vi "ExAppCamera.vi"() -> ()   [LabVIEW 2010]
uses:
  GlobalCamOpen.vi
  GlobalCCDMaxDim.vi
  GlobalInitializeFlag.vi
  GlobalFramesToStr.vi
  GlobalTimingMode.vi
  GlobalAcquireFocusFlag.vi
  GlobalExposure.vi
  GlobalUserBin.vi
  GlobalBin2x.vi
  GlobalFullBin.vi
  GlobalFlipFlag.vi
  GlobalReverseFlag.vi
  GlobalIBackImgHndl.vi
  GlobalIFlatImgHndl.vi
panel:
  out "Camera Opened":bool
  in  "Exit program":bool
  out "error out":errorcluster
  in  "error in (no error)":errorcluster
  in  "Tab Control":T1(tab)
  in  "Focus/Acquire Mode":u32=1 min=1 max=5 step=1
  in  "Number of Frames to store":u32=1 min=1 step=1
  in  "Intensifier":bool
  in  "Readout Port":i32=-1 min=-1 step=1
  in  "ADC Offset 2":i32=-1 min=-1 step=1
  in  "ADC Gain 2":i32=-1 min=-1 step=1
  in  "ADC speed":i32=-2 min=-3 step=1
  in  "Trigger Edge":u32(ring)=1 items=["N/A", "Positive (leading) edge", "Negative (falling) edge"]
  in  "Timing Mode":u32(ring)=1 items=["N/A", "Free Run/Timed", "Trigger First (PM only)", "Ext Sync/Strobed ", "Variable Exp (PM only)", "Flash Mode (PM only)"]
  out "Pixel Time":i32
  out "Bit Depth":i32
  out "ReadOut port":i32
  out "ADC Offset":i32
  out "ADC Gain":i32
  out "ADC Speed":i32
  in  "Set Experiment \nParameters, Initialize \nCamera/Controller":bool
  out "temperature":dbl format="%.2f"
  out "Temperature Read":dbl(slide) scale=-120.0..20.0
  in  "Temperature":dbl format="%.2f"
  in  "Exposure":dbl format="%.2f"
  out "Controller Initialized":bool
  out "Total":u32
  out "Y dim":u32
  out "X dim":u32
  in  "Y Bin":u32=1 min=1 step=1
  in  "Y End":u32=100 min=1 step=1
  in  "Y Start":u32=1 min=1 step=1
  in  "X Bin":u32=1 min=1 step=1
  in  "X End":u32=100 min=1 step=1
  in  "X Start":u32=1 min=1 step=1
  out "Bin 2":bool
  out "User":bool
  out "Full":bool
  in  "Binned by 2 Button":bool
  in  "User Defined Button":bool
  in  "Full CCD Button":bool
  out "Flip\nActive":bool
  in  "Flip flag Button":bool
  out "Reverse\nActive":bool
  in  "Image Reverse Button":bool
  out "Flat Field\nActive":bool
  out "Background \nActive":bool
  in  "Frame number to read":u32=1 min=1 step=1
  in  "Flat Button":bool
  in  "Back Button":bool
  in  "Full File Name":path
  in  "FileType":u32=67371008
  out "Reverse\nactive":bool
  out "Flip\nactive":bool
  out "Flat Field\nactive":bool
  out "background\nactive":bool
  in  "Reverse\nbutton":bool
  in  "Flip\nbutton":bool
  in  "Flat Field\nbutton":bool
  in  "Background\nbutton":bool
  in  "stop 2":bool
  in  "Start":bool
  out "Camera initialized":bool
  in  "Full File Name\nfor Acqure":path
  in  "OK Button":bool
  out "camera initialized":bool
  # "Note: In order for any parameters to change and be downloaded the initialize button must be hit."
  # "The following are read \nfrom camera after setting\nvalues to left.\n-1 value means it isn't \nsupported by camera."
  # "For Slowest ADC speed set this to -3\nFor Fastest ADC speed set this to -2\nTo use current ADC speed don't  hook up or use -1\notherwise put speed in as kHz"
  # "To use current gain don't hook up or set to -1"
  # "To use current gain don't hook up or set to -1"
  # "To use current gain don't hook up or set to -1"
  # "NOTE: if background subtraction and/or flat field are set, there are no \nchecks in this example for changes to the ROI."
  # "Pixels coming back\nfrom Camera"
  # "File Types:\nSPE = 67371008\nTIF   = 67174400\nPMI  = 67436544"
  # "Browse match pattern is set to *.spe.  Modify this if different file type is needed."
  # "Instructions:\nMake sure camera/controller has been initialized.  LED should be ON.\nPress \"Start Data collection\" button (a display should appear).\nWhen done press the \"STOP\" button (the display should disappear).\nLive Operation buttons only work while collecting data (not before)\nTo setup Live Operations before, go to Live Operations tab."
  # "Live Operations\n(will only work while collecting data)."
  # "Instructions:\nMake sure the camera/controller has been initialized (the light should be on).\nMake sure to put in a file name with path to save data.\nPress 'Start' button and display will pop up and data will be saved in file."
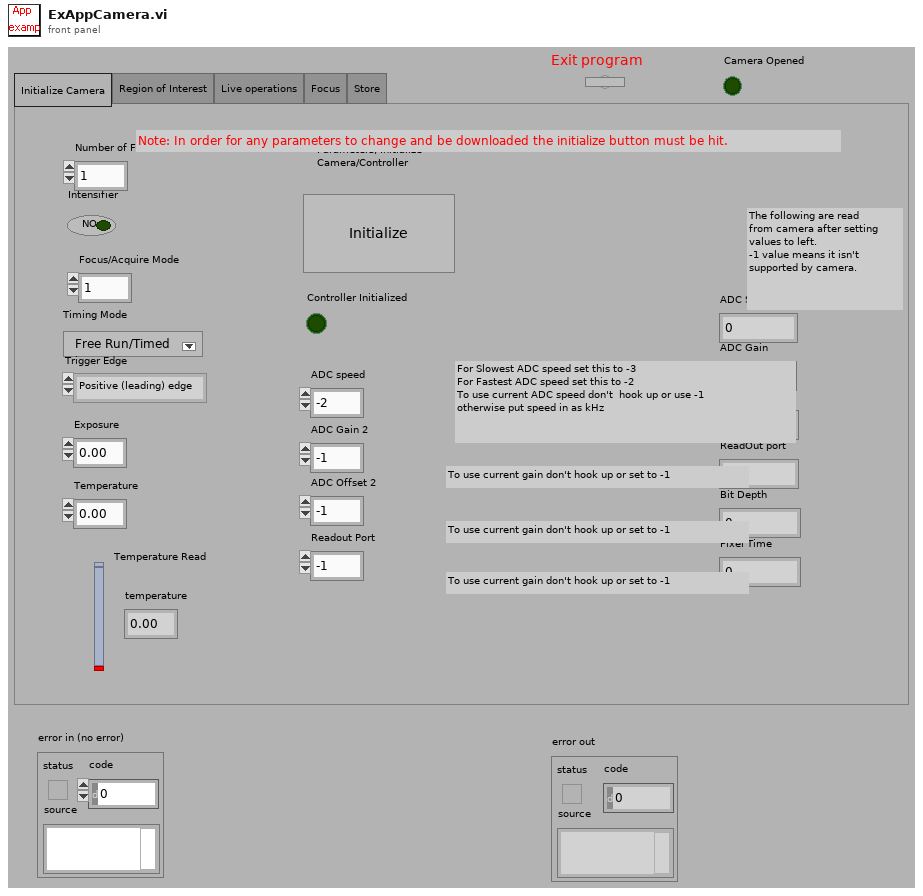
[diagram p1: front panel]
types:
  T1 = enum32{"Initialize Camera", "Region of Interest", "Live operations", "Focus", "Store"}
  T2 = cluster{"X Start":u32, "X End":u32, "X Bin":u32, "Y Start":u32, "Y End":u32, "Y Bin":u32}
  T3 = cluster{i32, "CCD Max X":u32, i32, i32, "CCD Max Y":u32, i32}
  T4 = cluster{"Camera Handle":u32, "Pulser Handle":u32, "File Handle":u32, "Display Handle":u32, "Image Handle":u32}
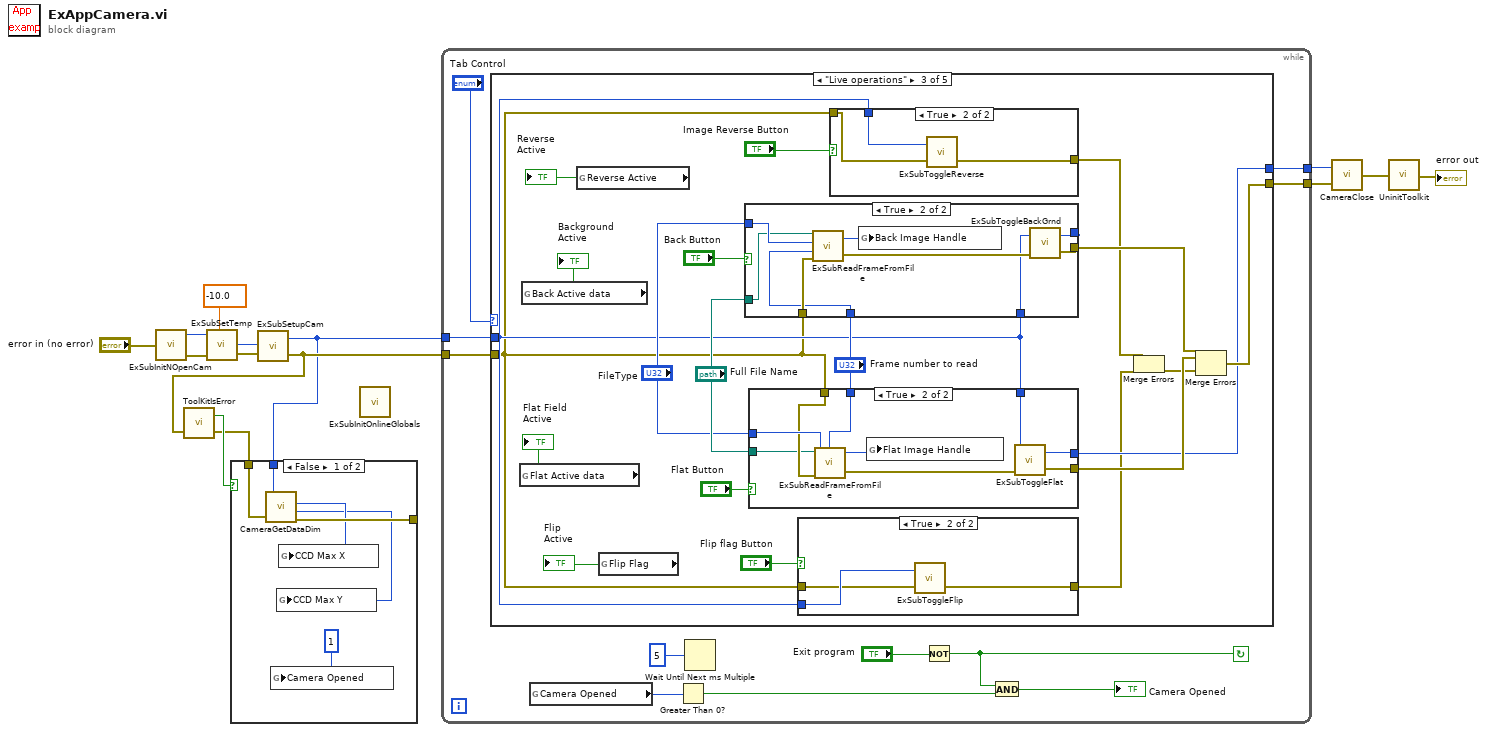
[diagram p0: block diagram]
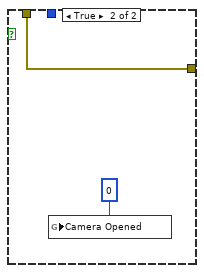
[diagram p2: hidden frame]
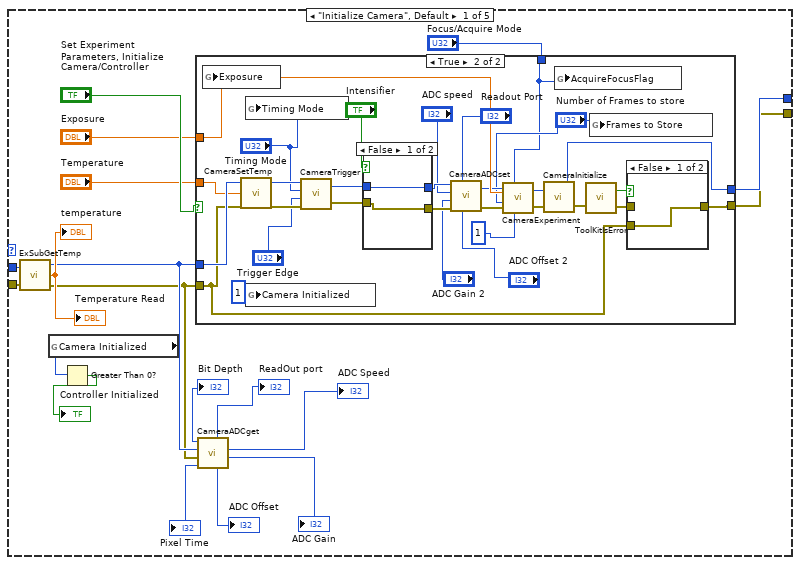
[diagram p3: hidden frame]
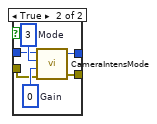
[diagram p6: hidden frame]
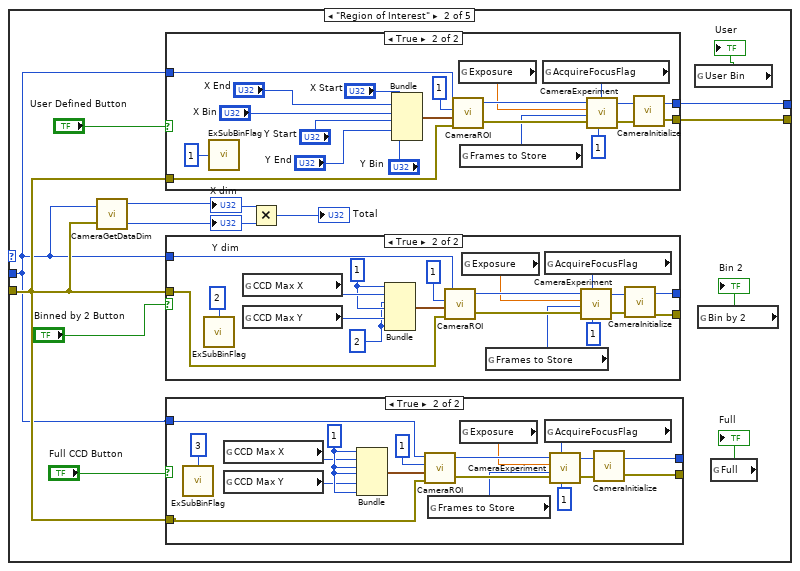
[diagram p7: hidden frame]
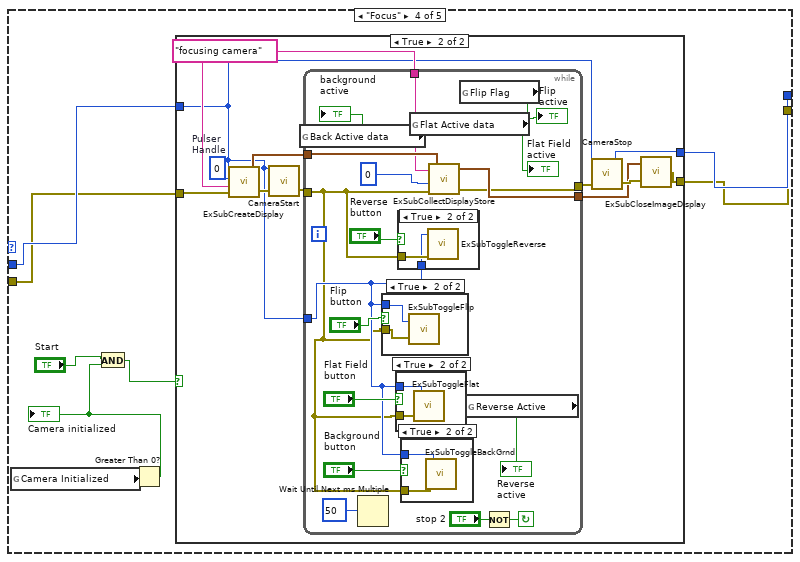
[diagram p15: hidden frame]
diagram:
  n1 = call "ExSubInitNOpenCam.vi"("error in (no error)"="error in (no error)") -> ("Camera Handle"=w12:u32, "error out"=w13:errorcluster)
  n2 = call "ExSubSetTemp.vi"("error in (no error)"=w13, "Temperature"=-10.0, "CameraHandle"=w12) -> ("error out"=w10:errorcluster, "Camera Handle"=w3:u32)
  n3 = call "ExSubSetupCam.vi"("error in (no error)"=w10, "Camera Handle"=w3) -> ("error out"=w4:errorcluster, "Camera Handle"=w2:u32)
  n4 = call <userlib>:"ToolKitIsError.vi"("error in"=w4) -> ("error out"=w1:errorcluster, "Error Flag"=w5:bool)  [unwired: 1 in]
  n5 = case shown="False" w5 {
    tunnel: w1 -> [w18 w22]
    tunnel: [w19 w22] -> _
    tunnel: w2 -> [w15 _]
    frame False {
      n6 = call <userlib>:"CameraGetDataDim.vi"("Camera Handle"=w15, "error in"=w18) -> ("Xdim"=w17:u32, "Ydim"=w16:u32, "error out"=w19:errorcluster)  [unwired: 1 out]
      n7 = global write "GlobalCamOpen.vi" "Camera Opened"(1) -> ()
      n8 = global write "GlobalCCDMaxDim.vi" "CCD Max Y"(w16) -> ()
      n9 = global write "GlobalCCDMaxDim.vi" "CCD Max X"(w17) -> ()
    }
    frame True {
      n10 = global write "GlobalCamOpen.vi" "Camera Opened"(0) -> ()
    }
  }
  n11 = call "ExSubInitOnlineGlobals.vi"() -> ()  [unwired: 1 in]
  n12 = while {
    tunnel: w2 -> [w33]
    tunnel: w4 -> [w30]
    tunnel: [w29] -> w9
    tunnel: [w28] -> w8
    stop <- w26 continue-if-true
    n13 = case shown="\"Live operations\"" "Tab Control" {
      tunnel: w33 -> [w52 w100 w176 w223 w273]
      tunnel: w30 -> [w44 w101 w175 w222 w272]
      tunnel: [w36 w99 w183 w225 w270] -> w29
      tunnel: [w35 w98 w184 w224 w271] -> w28
      frame "Initialize Camera", Default {
        n14 = call "ExSubGetTemp.vi"("Camera Handle"=w52, "error in (no error)"=w44) -> ("Camera Handle"=w43:u32, "Actual Temperature"=→"temperature" →"Temperature Read":dbl, "error out"=w42:errorcluster)
        n15 = global read "GlobalInitializeFlag.vi" "Camera Initialized"() -> (w47:u32)
        n16 = Greater Than 0?(x=w47) -> (x > 0?=→"Controller Initialized":bool)
        n17 = case shown="True" "Set Experiment \nParameters, Initialize \nCamera/Controller" {
          tunnel: "Exposure" -> [_ w73]
          tunnel: "Temperature" -> [_ w82]
          tunnel: w42 -> [w53 w57]
          tunnel: w43 -> [w54 w83]
          tunnel: [w53 w60] -> w35
          tunnel: [w54 w58] -> w36
          tunnel: "Focus/Acquire Mode" -> [_ w55]
          frame False {
          }
          frame True {
            n18 = global write "GlobalExposure.vi" "Exposure"(w73) -> ()
            n19 = call <userlib>:"CameraSetTemp.vi"("error in (no error)"=w57, "Temperature"=w82, "Camera Handle"=w83) -> ("error out"=w72:errorcluster, "Camera Handle"=w71:u32)
            n20 = global write "GlobalTimingMode.vi" "Timing Mode"("Timing Mode") -> ()
            n21 = global write "GlobalInitializeFlag.vi" "Camera Initialized"(1) -> ()
            n22 = call <userlib>:"CameraTrigger.vi"("error in"=w72, "Trigger Edge"="Trigger Edge", "Timing Mode"="Timing Mode", "Camera Handle"=w71) -> ("error out"=w68:errorcluster, "Camera Handle"=w69:u32)
            n23 = case shown="False" "Intensifier" {
              tunnel: [w88 w94] -> w79
              tunnel: [w87 w93] -> w80
              tunnel: w69 -> [w88 w90]
              tunnel: w68 -> [w87 w89]
              frame False {
              }
              frame True {
                w91 = u32 0  # Gain
                w92 = u32 3  # Mode
                n24 = call <userlib>:"CameraIntensMode.vi"("error in"=w89, "Intensifier Gain"=w91, "Mode"=w92, "Camera Handle"=w90) -> ("error out"=w93:errorcluster, "Camera Handle"=w94:u32)
              }
            }
            n25 = call <userlib>:"CameraADCset.vi"("ADC offset"="ADC Offset 2", "Read Out port"="Readout Port", "error in (no error)"=w80, "ADC Gain"="ADC Gain 2", "ADC Speed"="ADC speed", "Camera Handle"=w79) -> ("error out"=w66:errorcluster, "Camera Handle"=w65:u32)
            n26 = call <userlib>:"CameraExperiment.vi"("Number of Accumulations"=1, "Acquire / Focus Flag"=w55, "error in"=w66, "Number of Images"="Number of Frames to store", "Exposure (sec)"=w73, "Camera Handle"=w65) -> ("error out"=w64:errorcluster, "Camera Handle"=w63:u32)
            n27 = call <userlib>:"CameraInitialize.vi"("error in"=w64, "Camera Handle"=w63) -> ("error out"=w59:errorcluster, "Camera Handle"=w58:u32)
            n28 = global write "GlobalAcquireFocusFlag.vi" "AcquireFocusFlag"(w55) -> ()
            n29 = call <userlib>:"ToolKitIsError.vi"("error in"=w59) -> ("error out"=w61:errorcluster, "Error Flag"=w62:bool)  [unwired: 1 in]
            n30 = global write "GlobalFramesToStr.vi" "Frames to Store"("Number of Frames to store") -> ()
            n31 = case shown="False" w62 {
              tunnel: w61 -> [_ w86]
              tunnel: [w85 w86] -> w60
              tunnel: w57 -> [w85 _]
              frame False {
              }
              frame True {
              }
            }
          }
        }
        n32 = call <userlib>:"CameraADCget.vi"("Camera handle"=w43, "error in (no error)"=w42) -> ("Bit Depth"=→"Bit Depth":i32, "Pixel Time"=→"Pixel Time":i32, "Readout Port"=→"ReadOut port":i32, "ADC Offset"=→"ADC Offset":i32, "ADC Speed"=→"ADC Speed":i32, "ADC Gain"=→"ADC Gain":i32)  [unwired: 2 out]
      }
      frame "Region of Interest" {
        n33 = call <userlib>:"CameraGetDataDim.vi"("Camera Handle"=w100, "error in"=w101) -> ("Xdim"=w97:u32, "Ydim"=w96:u32)  [unwired: 2 out]
        "X dim" <- w97
        "Y dim" <- w96
        n34 = case shown="True" "User Defined Button" {
          tunnel: w100 -> [w150 w154]
          tunnel: [w150 w169] -> w99
          tunnel: w101 -> [w149 w153]
          tunnel: [w149 w166] -> w98
          frame False {
          }
          frame True {
            n35 = call "ExSubBinFlag.vi"("Binning \nUser = 1\nBin 2 = 2\nFull = 3"=1) -> ()
            n36 = Bundle("X Start"="X Start", "X End"="X End", "X Bin"="X Bin", "Y Start"="Y Start", "Y End"="Y End", "Y Bin"="Y Bin") -> (w155:T2)  [unwired: 1 in]
            n37 = call <userlib>:"CameraROI.vi"("error in"=w153, "ROI Params"=w155, "ROI Index"=1, "Camera Handle"=w154) -> ("error out"=w168:errorcluster, "Camera Handle"=w171:u32)
            n38 = global read "GlobalExposure.vi" "Exposure"() -> (w164:dbl)
            n39 = global read "GlobalFramesToStr.vi" "Frames to Store"() -> (w163:u32)
            n40 = global read "GlobalAcquireFocusFlag.vi" "AcquireFocusFlag"() -> (w162:u32)
            n41 = call <userlib>:"CameraExperiment.vi"("Number of Accumulations"=1, "Acquire / Focus Flag"=w162, "error in"=w168, "Number of Images"=w163, "Exposure (sec)"=w164, "Camera Handle"=w171) -> ("error out"=w167:errorcluster, "Camera Handle"=w170:u32)
            n42 = call <userlib>:"CameraInitialize.vi"("error in"=w167, "Camera Handle"=w170) -> ("error out"=w166:errorcluster, "Camera Handle"=w169:u32)
          }
        }
        n43 = case shown="True" "Binned by 2 Button" {
          tunnel: w100 -> [w129 w134]
          tunnel: [w129 w140] -> _
          tunnel: w101 -> [w128 w135]
          tunnel: [w128 w139] -> _
          frame False {
          }
          frame True {
            w131 = 2
            w132 = 1
            n44 = call "ExSubBinFlag.vi"("Binning \nUser = 1\nBin 2 = 2\nFull = 3"=2) -> ()
            n45 = global read "GlobalCCDMaxDim.vi" "CCD Max X"() -> (w138:u32)
            n46 = global read "GlobalCCDMaxDim.vi" "CCD Max Y"() -> (w137:u32)
            n47 = Bundle(w132, "CCD Max X"=w138, w131, w132, "CCD Max Y"=w137, w131) -> (w136:T3)  [unwired: 1 in]
            n48 = call <userlib>:"CameraROI.vi"("error in"=w135, "ROI Params"=w136, "ROI Index"=1, "Camera Handle"=w134) -> ("error out"=w146:errorcluster, "Camera Handle"=w148:u32)
            n49 = global read "GlobalExposure.vi" "Exposure"() -> (w143:dbl)
            n50 = global read "GlobalFramesToStr.vi" "Frames to Store"() -> (w142:u32)
            n51 = global read "GlobalAcquireFocusFlag.vi" "AcquireFocusFlag"() -> (w141:u32)
            n52 = call <userlib>:"CameraExperiment.vi"("Number of Accumulations"=1, "Acquire / Focus Flag"=w141, "error in"=w146, "Number of Images"=w142, "Exposure (sec)"=w143, "Camera Handle"=w148) -> ("error out"=w145:errorcluster, "Camera Handle"=w147:u32)
            n53 = call <userlib>:"CameraInitialize.vi"("error in"=w145, "Camera Handle"=w147) -> ("error out"=w139:errorcluster, "Camera Handle"=w140:u32)
          }
        }
        n54 = case shown="True" "Full CCD Button" {
          tunnel: w100 -> [w109 w112]
          tunnel: [w109 w119] -> _
          tunnel: w101 -> [w108 w111]
          tunnel: [w108 w118] -> _
          frame False {
          }
          frame True {
            w117 = 1
            n55 = call "ExSubBinFlag.vi"("Binning \nUser = 1\nBin 2 = 2\nFull = 3"=3) -> ()
            n56 = global read "GlobalCCDMaxDim.vi" "CCD Max X"() -> (w116:u32)
            n57 = global read "GlobalCCDMaxDim.vi" "CCD Max Y"() -> (w115:u32)
            n58 = Bundle(w117, "CCD Max X"=w116, w117, w117, "CCD Max Y"=w115, w117) -> (w114:T3)  [unwired: 1 in]
            n59 = call <userlib>:"CameraROI.vi"("error in"=w111, "ROI Params"=w114, "ROI Index"=1, "Camera Handle"=w112) -> ("error out"=w125:errorcluster, "Camera Handle"=w127:u32)
            n60 = global read "GlobalFramesToStr.vi" "Frames to Store"() -> (w121:u32)
            n61 = global read "GlobalExposure.vi" "Exposure"() -> (w122:dbl)
            n62 = global read "GlobalAcquireFocusFlag.vi" "AcquireFocusFlag"() -> (w120:u32)
            n63 = call <userlib>:"CameraExperiment.vi"("Number of Accumulations"=1, "Acquire / Focus Flag"=w120, "error in"=w125, "Number of Images"=w121, "Exposure (sec)"=w122, "Camera Handle"=w127) -> ("error out"=w124:errorcluster, "Camera Handle"=w126:u32)
            n64 = call <userlib>:"CameraInitialize.vi"("error in"=w124, "Camera Handle"=w126) -> ("error out"=w118:errorcluster, "Camera Handle"=w119:u32)
          }
        }
        n65 = Multiply(x=w97, y=w96) -> (x*y=→"Total":u32)
        n66 = global read "GlobalUserBin.vi" "User Bin"() -> (→"User":bool)
        n67 = global read "GlobalBin2x.vi" "Bin by 2"() -> (→"Bin 2":bool)
        n68 = global read "GlobalFullBin.vi" "Full"() -> (→"Full":bool)
      }
      frame "Live operations" {
        n69 = global read "GlobalIFlatImgHndl.vi" "Flat Active data"() -> (→"Flat Field\nActive":bool)
        n70 = global read "GlobalIBackImgHndl.vi" "Back Active data"() -> (→"Background \nActive":bool)
        n71 = global read "GlobalReverseFlag.vi" "Reverse Active"() -> (→"Reverse\nActive":bool)
        n72 = global read "GlobalFlipFlag.vi" "Flip Flag"() -> (→"Flip\nActive":bool)
        n73 = case shown="True" "Back Button" {
          tunnel: "Full File Name" -> [_ w219]
          tunnel: "FileType" -> [_ w220]
          tunnel: w175 -> [w212 w221]
          tunnel: [w212 w215] -> w186
          tunnel: "Frame number to read" -> [_ w218]
          tunnel: w176 -> [w211 w214]
          tunnel: [w211 w213] -> _
          frame False {
          }
          frame True {
            n74 = call "ExSubReadFrameFromFile.vi"("error in (no error)"=w221, "Frame to pull off"=w218, "File type"=w220, "path to file to open"=w219) -> ("error out"=w216:errorcluster, "Image Handle"=w217:u32)
            n75 = global write "GlobalIBackImgHndl.vi" "Back Image Handle"(w217) -> ()
            n76 = call "ExSubToggleBackGrnd.vi"("error in (no error)"=w216, "Camera Handle"=w214) -> ("error out"=w215:errorcluster, "Camera Handle"=w213:u32)
          }
        }
        n77 = case shown="True" "Flat Button" {
          tunnel: "Full File Name" -> [_ w207]
          tunnel: "FileType" -> [_ w210]
          tunnel: w175 -> [w201 w208]
          tunnel: [w201 w203] -> w185
          tunnel: "Frame number to read" -> [_ w209]
          tunnel: w176 -> [w200 w205]
          tunnel: [w200 w204] -> w183
          frame False {
          }
          frame True {
            n78 = call "ExSubReadFrameFromFile.vi"("error in (no error)"=w208, "Frame to pull off"=w209, "File type"=w210, "path to file to open"=w207) -> ("error out"=w202:errorcluster, "Image Handle"=w206:u32)
            n79 = global write "GlobalIFlatImgHndl.vi" "Flat Image Handle"(w206) -> ()
            n80 = call "ExSubToggleFlat.vi"("error in (no error)"=w202, "Camera Handle"=w205) -> ("error out"=w203:errorcluster, "Camera Handle"=w204:u32)
          }
        }
        n81 = case shown="True" "Flip flag Button" {
          tunnel: w176 -> [_ w199]
          tunnel: w175 -> [w196 w198]
          tunnel: [w196 w197] -> w174
          frame False {
          }
          frame True {
            n82 = call "ExSubToggleFlip.vi"("error in (no error)"=w198, "Camera Handle"=w199) -> ("error out"=w197:errorcluster)  [unwired: 1 out]
          }
        }
        n83 = case shown="True" "Image Reverse Button" {
          tunnel: w176 -> [_ w194]
          tunnel: w175 -> [w192 w195]
          tunnel: [w192 w193] -> w173
          frame False {
          }
          frame True {
            n84 = call "ExSubToggleReverse.vi"("error in (no error)"=w195, "Camera Handle"=w194) -> ("error out"=w193:errorcluster)  [unwired: 1 out]
          }
        }
        n85 = Merge Errors(w173, w174) -> (w172:errorcluster)
        n86 = Merge Errors(w186, w185, w172) -> (w184:errorcluster)
      }
      frame "Focus" {
        n87 = global read "GlobalInitializeFlag.vi" "Camera Initialized"() -> (w227:u32)
        n88 = Greater Than 0?(x=w227) -> (x > 0?=w226:bool)
        "Camera initialized" <- w226
        n89 = And(x="Start", y=w226) -> (x .and. y?=w229:bool)
        n90 = case shown="True" w229 {
          tunnel: w222 -> [w230 w239]
          tunnel: w223 -> [w231 w232]
          tunnel: [w231 w236] -> w225
          tunnel: [w230 w235] -> w224
          frame False {
          }
          frame True {
            w233 = "focusing camera"
            w240 = u32 0  # Pulser  Handle
            n91 = call "ExSubCreateDisplay.vi"("error in (no error)"=w239, "File and Display Name"=w233, "Pulser Handle"=w240, "Camera Handle"=w232) -> ("error out"=w241:errorcluster, "Handles Out"=w243:T4)
            n92 = call <userlib>:"CameraStart.vi"("error in"=w241, "Camera Handle"=w232) -> ("error out"=w242:errorcluster)  [unwired: 1 out]
            n93 = while {
              tunnel: w243 -> [w260]
              tunnel: w242 -> [w248]
              tunnel: [w258] -> w238
              tunnel: [w259] -> w234
              tunnel: w233 -> [w254]
              tunnel: w232 -> [w249]
              stop <- w256 continue-if-true
              n94 = global read "GlobalIBackImgHndl.vi" "Back Active data"() -> (→"background\nactive":bool)
              n95 = Wait Until Next ms Multiple(millisecond multiple=u32 50) -> ()  [unwired: 1 out]
              n96 = case shown="True" "Flip\nbutton" {
                tunnel: w249 -> [_ w266]
                tunnel: w248 -> [_ w267]
                frame False {
                }
                frame True {
                  n97 = call "ExSubToggleFlip.vi"("error in (no error)"=w267, "Camera Handle"=w266) -> ()  [unwired: 2 out]
                }
              }
              n98 = case shown="True" "Flat Field\nbutton" {
                tunnel: w249 -> [_ w264]
                tunnel: w248 -> [_ w265]
                frame False {
                }
                frame True {
                  n99 = call "ExSubToggleFlat.vi"("error in (no error)"=w265, "Camera Handle"=w264) -> ()  [unwired: 2 out]
                }
              }
              n100 = case shown="True" "Reverse\nbutton" {
                tunnel: w248 -> [_ w269]
                tunnel: w249 -> [_ w268]
                frame False {
                }
                frame True {
                  n101 = call "ExSubToggleReverse.vi"("error in (no error)"=w269, "Camera Handle"=w268) -> ()  [unwired: 2 out]
                }
              }
              n102 = case shown="True" "Background\nbutton" {
                tunnel: w249 -> [_ w263]
                tunnel: w248 -> [_ w262]
                frame False {
                }
                frame True {
                  n103 = call "ExSubToggleBackGrnd.vi"("error in (no error)"=w262, "Camera Handle"=w263) -> ()  [unwired: 2 out]
                }
              }
              n104 = global read "GlobalIFlatImgHndl.vi" "Flat Active data"() -> (→"Flat Field\nactive":bool)
              n105 = call "ExSubCollectDisplayStore.vi"("error in (no error)"=w248, "Store flag"=0, "Display Title"=w254, "Handle Cluster"=w260) -> ("error out"=w258:errorcluster, "Handle Cluster Out"=w259:T4)  [unwired: 1 out]
              n106 = global read "GlobalFlipFlag.vi" "Flip Flag"() -> (→"Flip\nactive":bool)
              n107 = global read "GlobalReverseFlag.vi" "Reverse Active"() -> (→"Reverse\nactive":bool)
              n108 = Not(x="stop 2") -> (.not. x?=w256:bool)
            }
            n109 = call <userlib>:"CameraStop.vi"("error in"=w238, "Camera Handle"=w232) -> ("error out"=w237:errorcluster, "Camera Handle"=w236:u32)
            n110 = call "ExSubCloseImageDisplay.vi"("error in (no error)"=w237, "Handles In"=w234) -> ("error out"=w235:errorcluster)
          }
        }
      }
      frame "Store" {
        n111 = global read "GlobalInitializeFlag.vi" "Camera Initialized"() -> (w275:u32)
        n112 = Greater Than 0?(x=w275) -> (x > 0?=w274:bool)
        "camera initialized" <- w274
        n113 = And(x="OK Button", y=w274) -> (x .and. y?=w277:bool)
        n114 = case shown="True" w277 {
          tunnel: w273 -> [w279 w288]
          tunnel: w272 -> [w278 w289]
          tunnel: [w278 w280] -> w271
          tunnel: [w279 w288] -> w270
          frame False {
          }
          frame True {
            w292 = u32 0  # Pulser Handle
            n115 = Path To String(path="Full File Name\nfor Acqure") -> (string=w290:string)
            n116 = global read "GlobalFramesToStr.vi" "Frames to Store"() -> (w282:u32)
            n117 = call "ExSubCreateFileDisplay.vi"("error in (no error)"=w289, "File and Display Name"=w290, "Pulser Handle"=w292, "Camera Handle"=w288) -> ("error out"=w293:errorcluster, "Handles Out"=w283:T4)
            n118 = call <userlib>:"CameraStart.vi"("error in"=w293, "Camera Handle"=w288) -> ("error out"=w284:errorcluster, "Camera Handle"=w281:u32)
            n119 = call "ExSubNframeCol.vi"("error in (no error)"=w284, "Number of Images"=w282, "Handle Cluster"=w283) -> ("error out"=w287:errorcluster, "Handle Cluster"=w286:T4)
            n120 = call <userlib>:"CameraStop.vi"("error in"=w287, "Camera Handle"=w281) -> ("error out"=w285:errorcluster)  [unwired: 1 out]
            n121 = call "ExSubCloseFileImageDisplay.vi"("error in (no error)"=w285, "Handles In"=w286) -> ("error out"=w280:errorcluster)
          }
        }
      }
    }
    n122 = global read "GlobalCamOpen.vi" "Camera Opened"() -> (w27:u32)
    n123 = Greater Than 0?(x=w27) -> (x > 0?=w25:bool)
    n124 = Wait Until Next ms Multiple(millisecond multiple=5) -> ()  [unwired: 1 out]
    n125 = Not(x="Exit program") -> (.not. x?=w26:bool)
    n126 = And(x=w26, y=w25) -> (x .and. y?=→"Camera Opened":bool)
  }
  n127 = call <userlib>:"CameraClose.vi"("error in"=w8, "Camera Handle"=w9) -> ("error out"=w7:errorcluster)
  n128 = call <userlib>:"UninitToolkit.vi"("error in"=w7) -> ("error out"=→"error out":errorcluster)
